vi "Hash.vi"(11 "in":string) -> (3 "out":string)   [LabVIEW 2020, in "hse-misc.lvlib"]
doc: "____\nHAMPEL SOFTWARE ENGINEERING v3.8.0 (2023-12-18 14:41)"
uses:
  hse-misc.lvlib
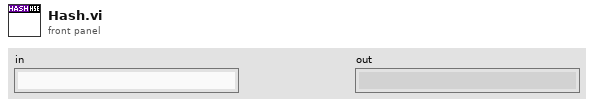
[diagram p1: front panel]
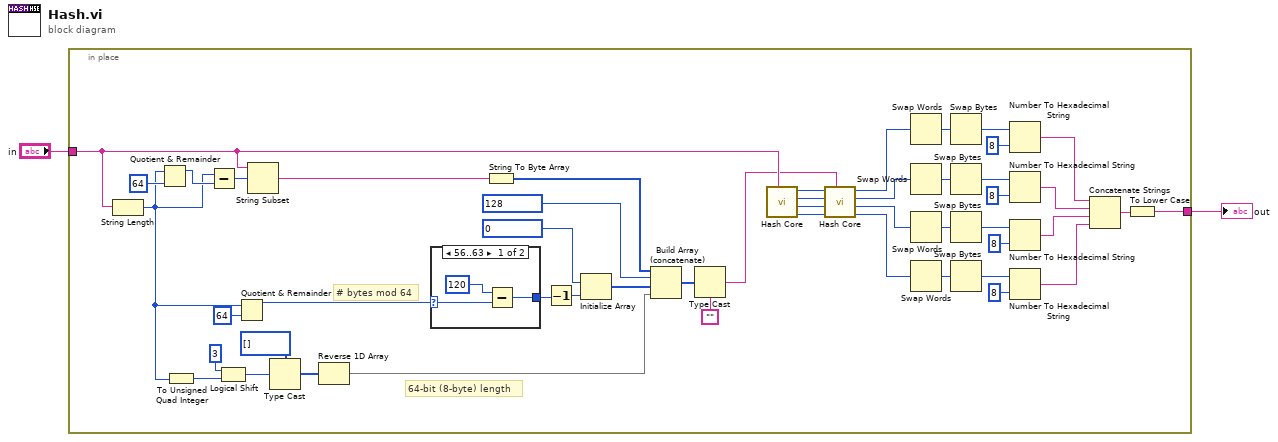
[diagram p0: block diagram]
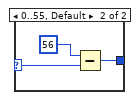
[diagram p2: hidden frame]
diagram:
  n1 = in-place {
    in-place-border: "in" -> [w51]
    in-place-border: [w50] -> w1
    # "64-bit (8-byte) length"
    # "# bytes mod 64"
    n2 = String Length(string=w51) -> (length=w4:i32)
    n3 = Quotient & Remainder(x=w4, y=64) -> (x-y*floor(x/y)=w43:i32)  [unwired: 1 out]
    n4 = To Unsigned Quad Integer(1:w4) -> (0:w10:u64)
    n5 = Subtract(x=w4, y=w43) -> (x-y=w44:i32)
    n6 = Logical Shift(y=i16 3, x=w10) -> (x << y=w8:u64)
    n7 = Quotient & Remainder(x=w4, y=i64 64) -> (x-y*floor(x/y)=w13:i64)  [unwired: 1 out]
    n8 = String Subset(string=w51, offset (0)=w44) -> (substring=w5:string)  [unwired: 1 in]
    n9 = Type Cast(type=u8[] [], x=w8) -> (*(type *) &x=w7:u8[])
    n10 = Reverse 1D Array(array=w7) -> (reversed array=w6:u8[])
    n11 = case shown="56..63" w13 {
      selector: w13 -> [w53 w56]
      tunnel: [w52 w55] -> w15
      frame 56..63 {
        n12 = Subtract(x=i64 120, y=w53) -> (x-y=w52:i64)
      }
      frame 0..55, Default {
        n13 = Subtract(x=i64 56, y=w56) -> (x-y=w55:i64)
      }
    }
    n14 = String To Byte Array(string=w5) -> (unsigned byte array=w14:u8[])
    n15 = Decrement(x=w15) -> (x-1=w16:i64)
    n16 = Initialize Array(u8 0, w16) -> (w20:u8[])
    n17 = Build Array (concatenate)(w14, u8 128, w20, w6) -> (w17:u8[])
    n18 = Type Cast(type="", x=w17) -> (*(type *) &x=w3:string)
    n19 = call "Hash Core.vi"("Input String"=w51) -> ("s4 out"=w46:u32, "s3 out"=w47:u32, "s2 out"=w48:u32, "s1 out"=w49:u32)  [unwired: 6 in, 1 out]
    n20 = call "Hash Core.vi"("Input String"=w3, "s4 in"=w46, "s3 in"=w47, "s2 in"=w48, "s1 in"=w49) -> ("s4 out"=w22:u32, "s3 out"=w23:u32, "s2 out"=w24:u32, "s1 out"=w25:u32)  [unwired: 2 in, 1 out]
    n21 = Swap Words(1:w25) -> (0:w41:u32)
    n22 = Swap Words(1:w24) -> (0:w38:u32)
    n23 = Swap Words(1:w23) -> (0:w35:u32)
    n24 = Swap Words(1:w22) -> (0:w32:u32)
    n25 = Swap Bytes(anything=w41) -> (byte swapped=w40:u32)
    n26 = Swap Bytes(anything=w38) -> (byte swapped=w39:u32)
    n27 = Swap Bytes(anything=w35) -> (byte swapped=w34:u32)
    n28 = Swap Bytes(anything=w32) -> (byte swapped=w33:u32)
    n29 = Number To Hexadecimal String(1:i16 8 ("width (-)"), 2:w40) -> (0:w30:string)
    n30 = Number To Hexadecimal String(1:i16 8 ("width (-)"), 2:w39) -> (0:w29:string)
    n31 = Number To Hexadecimal String(1:i16 8 ("width (-)"), 2:w34) -> (0:w28:string)
    n32 = Number To Hexadecimal String(1:i16 8 ("width (-)"), 2:w33) -> (0:w27:string)
    n33 = Concatenate Strings(w30, w29, w28, w27) -> (w26:string)
    n34 = To Lower Case(string=w26) -> (all lower case string=w50:string)
  }
  "out" <- w1
